vi "Draw Expanded Values.vi"(4 "Expanded Types":T1[](array[typedef]), 6 "State":T7, 7 "Sizes":T6, 11 "Picture  In":picture) -> (3 "Picture":picture)   [LabVIEW 2020, in "FlexBlock.xnode"]
uses:
  FlexBlock.xnode
  State.ctl
  FlexBlocks/Type Descriptor.ctl
  FlexBlocks/Terminal Direction.ctl
  FlexBlocks/Value Mode.ctl
  FlexBlocks/Terminal State.ctl
  FlexBlocks/Special Terminal.ctl
  FlexBlocks/Errors.ctl
  <vilib>/picture/picture.llb/imagedata.ctl
  FlexBlocks/Calculated Sizes.ctl
  FlexBlocks/Size Constants.ctl
  FlexBlocks/FlexBlocks.lvlib
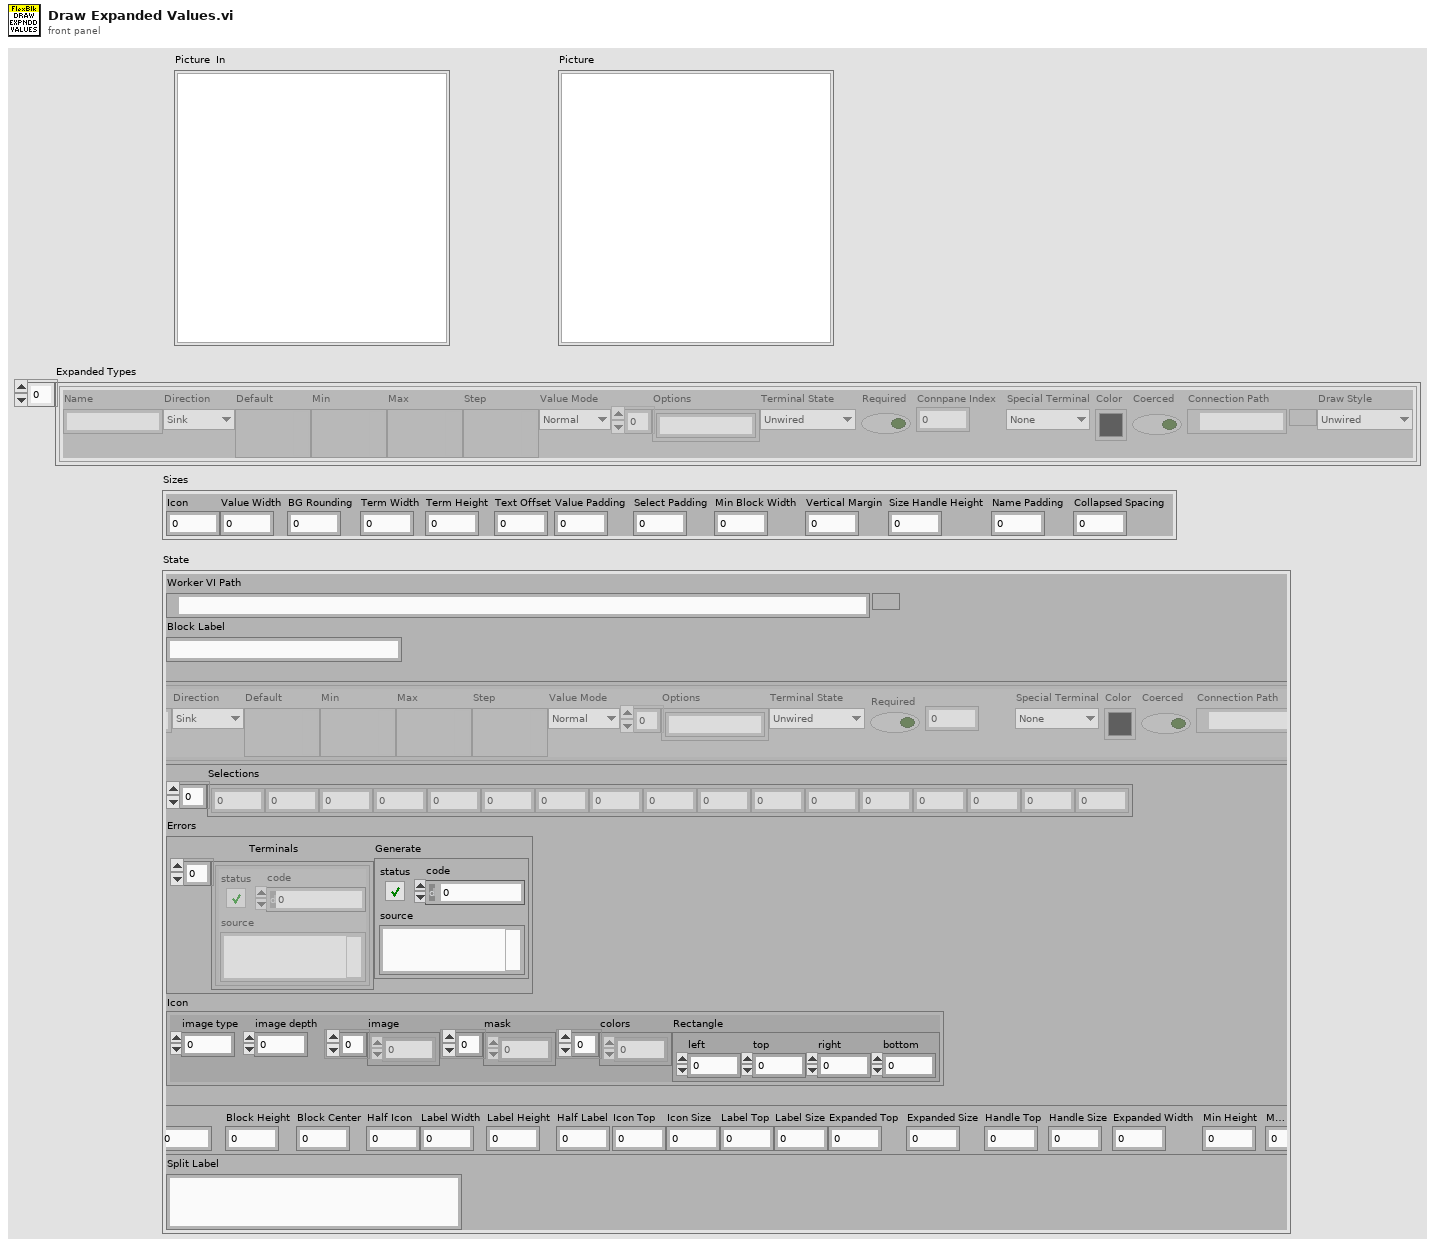
[diagram p1: front panel]
types:
  T1 = typedef "FlexBlocks.lvlib/Type Descriptor.ctl" = cluster{"Name":string, "Direction":T2, "Default":variant, "Min":variant, "Max":variant, "Step":variant, "Value Mode":T3, "Options":string[], "Terminal State":T4, "Required":bool, "Connpane Index":i32, "Special Terminal":T5, "Color":u32, "Coerced":bool, "Connection Path":path, "Draw Style":T4}
  T2 = typedef "FlexBlocks.lvlib/Terminal Direction.ctl" = enum16{"Sink", "Source"}
  T3 = typedef "FlexBlocks.lvlib/Value Mode.ctl" = enum16{"Normal", "Range", "Select"}
  T4 = typedef "FlexBlocks.lvlib/Terminal State.ctl" = enum16{"Unwired", "BadType", "BadRef", "Channel", "Value", "Control Ref"}
  T5 = typedef "FlexBlocks.lvlib/Special Terminal.ctl" = enum16{"None", "Action", "Init", "Tag", "State in", "State out", "Error"}
  T6 = typedef "FlexBlocks.lvlib/Size Constants.ctl" = cluster{"Icon":i32, "Value Width":i32, "BG Rounding":i32, "Term Width":i32, "Term Height":i32, "Text Offset":i32, "Value Padding":i32, "Select Padding":i32, "Min Block Width":i32, "Vertical Margin":i32, "Size Handle Height":i32, "Name Padding":i32, "Collapsed Spacing":i32}
  T7 = typedef "FlexBlock.xnode/State.ctl" = cluster{"Worker VI Path":path, "Block Label":string, "Types":T1[], "Selections":i32[], "Errors":T8, "Icon":T9, "Calcd Sizes":T10, "Split Label":string}
  T8 = typedef "FlexBlocks.lvlib/Errors.ctl" = cluster{"Terminals":errorcluster[], "Generate":errorcluster}
  T9 = typedef "imagedata.ctl" = cluster{"image type":i32, "image depth":i32, "image":u8[], "mask":u8[], "colors":u32[], "Rectangle":cluster{"left":i16, "top":i16, "right":i16, "bottom":i16}}
  T10 = typedef "FlexBlocks.lvlib/Calculated Sizes.ctl" = cluster{"Text Width":i32, "Text Height":i32, "Half Text":i32, "Block Width":i32, "Block Height":i32, "Block Center":i32, "Half Icon":i32, "Label Width":i32, "Label Height":i32, "Half Label":i32, "Icon Top":i32, "Icon Size":i32, "Label Top":i32, "Label Size":i32, "Expanded Top":i32, "Expanded Size":i32, "Handle Top":i32, "Handle Size":i32, "Expanded Width":i32, "Min Height":i32, "Max Height":i32}
  T11 = cluster{"left":i16, "top":i16, "right":i16, "bottom":i16}
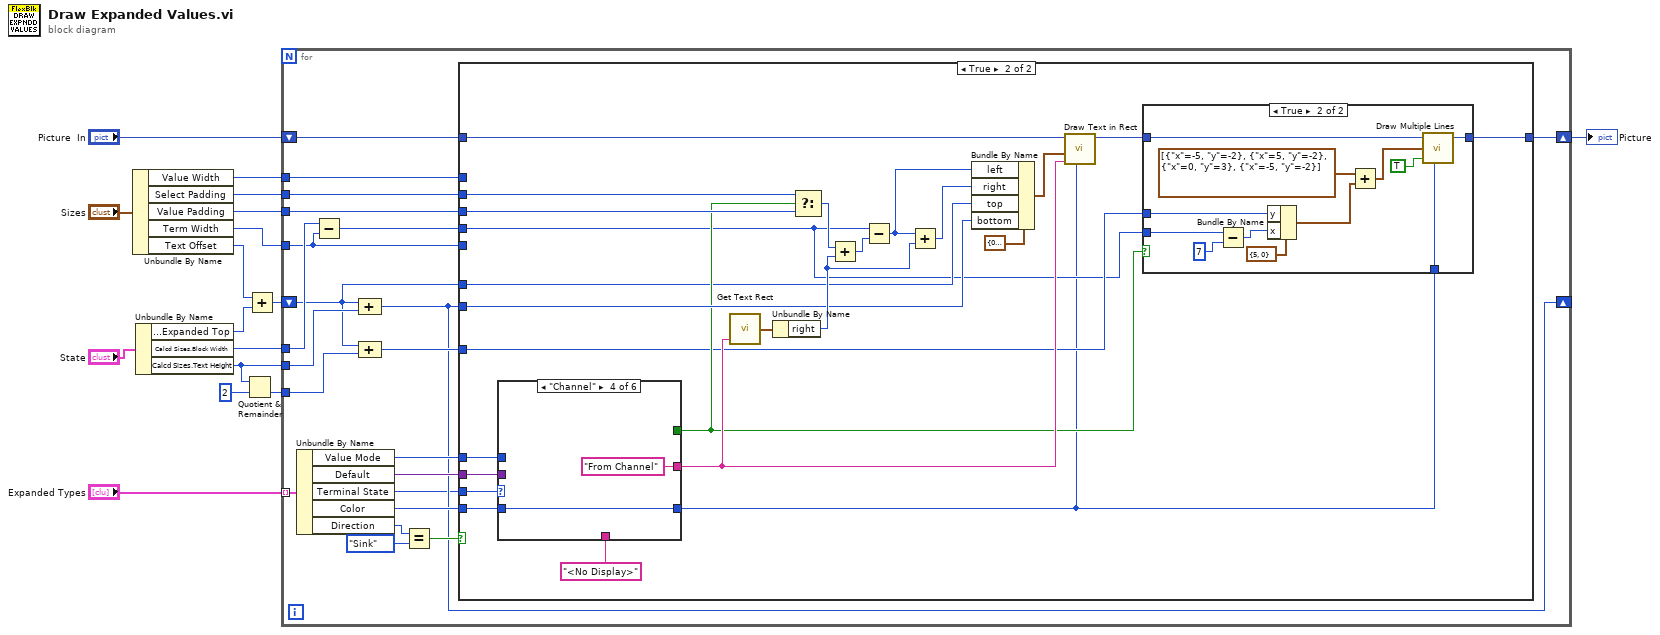
[diagram p0: block diagram]
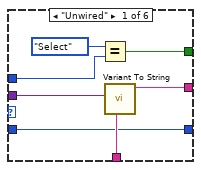
[diagram p3: hidden frame]
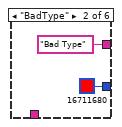
[diagram p4: hidden frame]
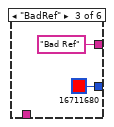
[diagram p5: hidden frame]
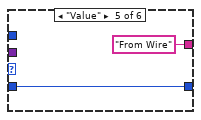
[diagram p6: hidden frame]
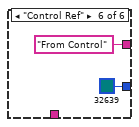
[diagram p7: hidden frame]
diagram:
  n1 = Unbundle By Name("Sizes") -> ("Value Width"=w1:i32, "Select Padding"=w6:i32, "Value Padding"=w7:i32, "Term Width"=w10:i32, "Text Offset"=w13:i32)
  n2 = Unbundle By Name("State") -> ("Calcd Sizes.Expanded Top"=w14:i32, "Calcd Sizes.Block Width"=w8:i32, "Calcd Sizes.Text Height"=w3:i32)
  n3 = Quotient & Remainder(x=w3, y=2) -> (floor(x/y)=w2:i32)  [unwired: 1 out]
  n4 = Add(x=w13, y=w14) -> (x+y=w9:i32)
  n5 = for {
    tunnel: "Expanded Types" -> [w37] mode=indexing
    tunnel: w10 -> [w19]
    shift-right: [w20] -> _
    shift-left: w9 -> [w26]
    tunnel: w8 -> [w29]
    tunnel: w3 -> [w34]
    tunnel: w7 -> [w32]
    tunnel: w6 -> [w31]
    shift-right: [w30] -> w5
    shift-left: "Picture  In" -> [w35]
    tunnel: w2 -> [w27]
    tunnel: w1 -> [w18]
    n6 = Unbundle By Name(w37) -> ("Value Mode"=w33:T3, "Default"=w36:variant, "Terminal State"=w17:T4, "Color"=w24:u32, "Direction"=w23:T2)
    n7 = Subtract(x=w29, y=w19) -> (x-y=w28:i32)
    n8 = Compound Arithmetic op=ADD(w26, w34) -> (w20:i32)
    n9 = Compound Arithmetic op=ADD(w26, w27) -> (w25:i32)
    n10 = Equal?(x=w23, y=Terminal_Direction."Sink") -> (x = y?=w21:bool)
    n11 = case shown="True" w21 {
      tunnel: w36 -> [_ w62]
      tunnel: w35 -> [w38 w60]
      tunnel: w33 -> [_ w56]
      tunnel: w32 -> [_ w55]
      tunnel: w31 -> [_ w54]
      tunnel: w20 -> [_ w48]
      tunnel: [w38 w46] -> w30
      tunnel: w28 -> [_ w42]
      tunnel: w26 -> [_ w44]
      tunnel: w25 -> [_ w43]
      tunnel: w24 -> [_ w41]
      tunnel: w19 -> [_ _]
      tunnel: w18 -> [_ _]
      tunnel: w17 -> [_ w40]
      frame False {
      }
      frame True {
        n12 = case shown="\"Channel\"" w40 {
          tunnel: "<No Display>" ("Unsupported (Empty)") -> [w70 _ _ _ _ _]
          tunnel: w62 -> [w69 _ _ _ _ _]
          tunnel: [w68 "Bad Type" ("String") "Bad Ref" ("String") "From Channel" ("String") "From Wire" ("String") "From Control" ("String")] -> w58
          tunnel: w56 -> [w67 _ _ _ _ _]
          tunnel: [w65 _ _ _ _ _] -> w45
          tunnel: w41 -> [w64 _ _ w75 w77 _]
          tunnel: [w64 u32 16711680 ("Color") u32 16711680 ("Color") w75 w77 u32 32639 ("Color")] -> w39
          frame "Unwired" {
            n13 = Equal?(x=Value_Mode."Select", y=w67) -> (x = y?=w65:bool)
            n14 = call "Variant To String.vi"("Unsupported (Empty)"=w70, "Variant"=w69) -> ("String"=w68:string)  [unwired: 8 in, 1 out]
          }
          frame "BadType" {
          }
          frame "BadRef" {
          }
          frame "Channel" {
          }
          frame "Value" {
          }
          frame "Control Ref" {
          }
        }
        n15 = call <vilib>:"Get Text Rect.vi"("text"=w58) -> ("rect"=w61:T11)  [unwired: 8 in]
        n16 = Unbundle By Name(w61) -> ("right"=w50:i16)
        n17 = Select(t=w54, s=w45, f=w55) -> (s? t:f=w53:i32)
        n18 = Add(x=w53, y=w50) -> (x+y=w52:i32)
        n19 = Subtract(x=w42, y=w52) -> (x-y=w51:i32)
        n20 = Add(x=w51, y=w50) -> (x+y=w49:i32)
        n21 = Bundle By Name(cluster=T11 {"left"=0, "top"=0, "right"=0, "bottom"=0} ("rect"), "left"=w51, "right"=w49, "top"=w44, "bottom"=w48) -> (w57:T11)
        n22 = call <vilib>:"Draw Text in Rect.vi"("text color(black)"=w39, "text"=w58, "rect"=w57, "picture"=w60) -> ("new picture"=w47:picture)  [unwired: 7 in]
        n23 = case shown="True" w45 {
          tunnel: w47 -> [w81 w93]
          tunnel: [w81 w92] -> w46
          tunnel: w43 -> [_ w86]
          tunnel: w42 -> [_ w83]
          tunnel: w39 -> [_ w82]
          frame False {
            # "Already fully expanded"
          }
          frame True {
            n24 = Subtract(x=w83, y=i16 7 ("x")) -> (x-y=w85:i32)
            n25 = Bundle By Name(cluster=cluster{"x":i16, "y":i16} {"x"=5, "y"=0}, "y"=w86, "x"=w85) -> (w89:cluster{"x":i16, "y":i16})
            n26 = Add(x=cluster{"x":i16, "y":i16}[] [{"x"=-5, "y"=-2}, {"x"=5, "y"=-2}, {"x"=0, "y"=3}, {"x"=-5, "y"=-2}] ("line endpoints"), y=w89) -> (x+y=w88:cluster{"x":i16, "y":i16}[])
            n27 = call <vilib>:"Draw Multiple Lines.vi"("picture"=w93, "line endpoints"=w88, "fill?(F)"=TRUE, "color(black)"=w82) -> ("new picture"=w92:picture)  [unwired: 5 in]
          }
        }
      }
    }
  }
  "Picture" <- w5
